vi "Teleop.vi"(10 "Match Info":T1={"Autonomous Elapsed Seconds"=0.0, "TeleOp Elapsed Seconds"=0.0, "Disabled Elapsed Seconds"=0.0, "Visited Autonomous"=FALSE, "Visited TeleOp"=FALSE, "Visited Disabled"=FALSE, "Autonomous Settings"={"Autonomous Style"=enum."Independent", "VI Refnum"=refnum}}, 11 "Call Context":T2) -> ()   [LabVIEW 2020]
doc: "This VI is called for each TeleOp packet received from the DS where the robot is not disabled. It is often used to read from the joysticks and update I/O or to update setpoints for timed control loops. It should complete and return within 20 milliseconds or it may miss DS packets."
uses:
  <vilib>/Rock Robotics/WPI/DriverStation/WPI_DriverStationDerivedRobotMode.ctl
  <vilib>/Rock Robotics/WPI/DriverStation/WPI_DriverStationMatch Info.ctl
  <vilib>/Rock Robotics/WPI/Utilities/WPI_GetSetVariantRefNum.vi
  <vilib>/Rock Robotics/Network Tables/NT Read Boolean.vi
  <vilib>/Rock Robotics/Network Tables/NT Read Number.vi
  Variable BX.vi
  RX.vi
  LX.vi
panel:
  out "Sample Slider 0":dbl(slide) scale=0.0..5.0
  out "Sample Boolean 1":bool
  out "Sample Boolean 0":bool
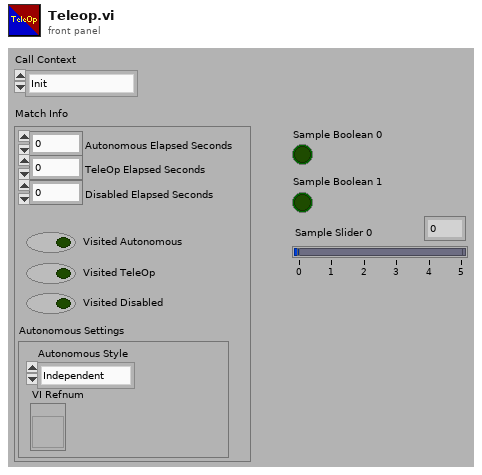
[diagram p1: front panel]
types:
  T1 = typedef "WPI_DriverStationMatch Info.ctl" = cluster{"Autonomous Elapsed Seconds":dbl, "TeleOp Elapsed Seconds":dbl, "Disabled Elapsed Seconds":dbl, "Visited Autonomous":bool, "Visited TeleOp":bool, "Visited Disabled":bool, "Autonomous Settings":cluster{"Autonomous Style":enum16{"Iterative", "Independent"}, "VI Refnum":refnum<vi>}}
  T2 = typedef "WPI_DriverStationDerivedRobotMode.ctl" = enum16{"Init", "Execute", "Stop"}
  T3 = typedef "WPI_MotorControlDeviceRef.ctl" = cluster{"DeviceStatus":errorcluster, "Type":T4, "PWM":cluster{"PWM Channel":T5, "DeadBand":T6}, "CAN":cluster{"Device Number":u8, "SetOutput VI Ref":variant, "GetOutput VI Ref":variant, "Enable VI Ref":variant, "Disable VI Ref":variant, "Data":variant}, "Invert":bool, "DIO PWM":cluster{"PWM \"Enable\" Channel":T5, "DIOChannel":T7, "PWM Rate":dbl}}
  T4 = typedef "WPI_MotorControlType.ctl" = enum16{"PWM", "CAN", "DIO PWM"}
  T5 = typedef "FPGA_DIOPWMChannel.ctl" = enum8{"PWM 0", "PWM 1", "PWM 2", "PWM 3", "PWM 4", "PWM 5", "PWM 6", "PWM 7", "PWM 8", "PWM 9", "PWM MXP 0", "PWM MXP 1", "PWM MXP 2", "PWM MXP 3", "PWM MXP 4", "PWM MXP 5", "PWM MXP 6", "PWM MXP 7", "PWM MXP 8", "PWM MXP 9", "Invalid"}
  T6 = typedef "WPI_PWMDeadband.ctl" = cluster{"Name":string, "maxPositivePwm":i32, "minPositivePwm":i32, "centerPwm":i32, "maxNegativePwm":i32, "minNegativePwm":i32, "angularRange":u16}
  T7 = typedef "FPGA_DIOChannel.ctl" = enum8{"DIO 0", "DIO 1", "DIO 2", "DIO 3", "DIO 4", "DIO 5", "DIO 6", "DIO 7", "DIO 8", "DIO 9", "DIO MXP 0", "DIO MXP 1", "DIO MXP 2", "DIO MXP 3", "DIO MXP 4", "DIO MXP 5", "DIO MXP 6", "DIO MXP 7", "DIO MXP 8", "DIO MXP 9", "DIO MXP 10", "DIO MXP 11", "DIO MXP 12", "DIO MXP 13", "DIO MXP 14", "DIO MXP 15", "SPI Port CS1", "SPI Port CS2", "SPI Port CS3", "SPI Port MISO", "SPI Port MOSI", "Invalid"}
  T8 = typedef "WPI_JoystickDevRef.ctl" = cluster{"Device":T9}
  T9 = typedef "WPI_JoystickDeviceEnum.ctl" = enum16{"USB 0", "USB 1", "USB 2", "USB 3", "USB 4", "USB 5"}
  T10 = typedef "WPI_RobotDriveDevRef.ctl" = cluster{"DevStatus":errorcluster, "Motors[]":T3[], "Square Inputs":bool, "Max Output":dbl}
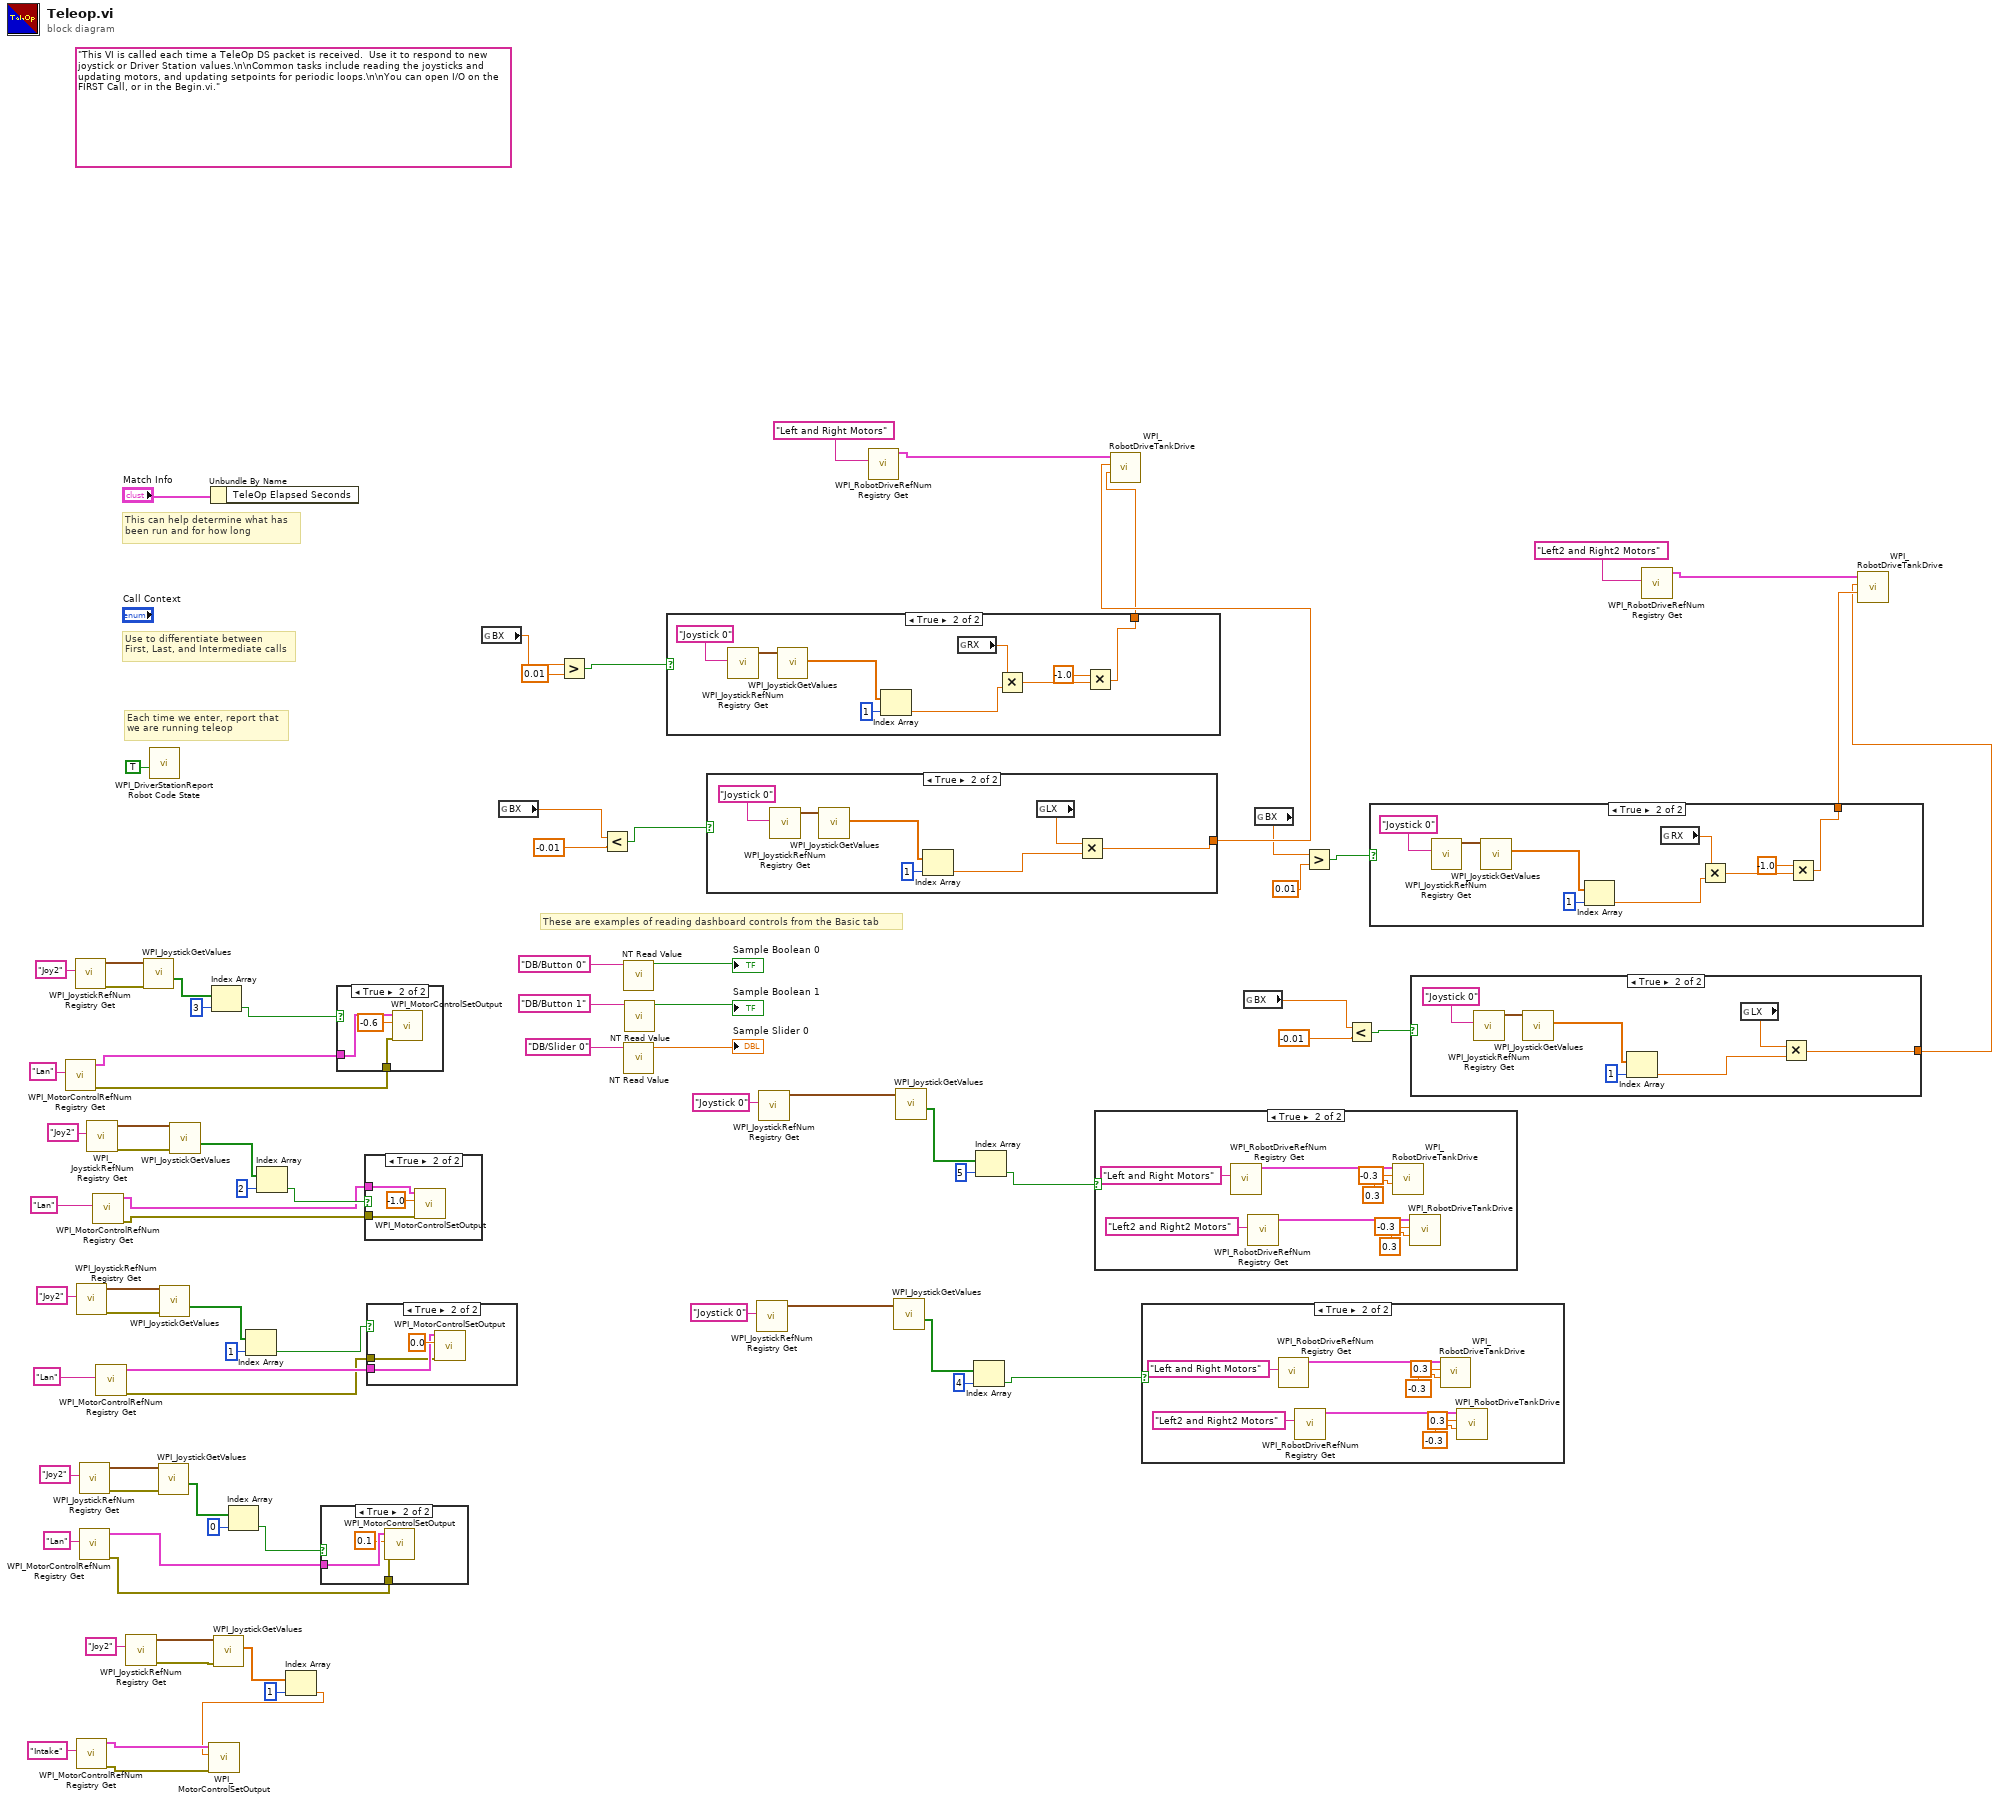
[diagram p0: block diagram]
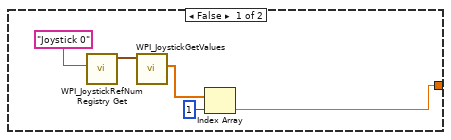
[diagram p8: hidden frame]
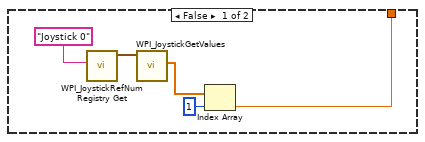
[diagram p9: hidden frame]
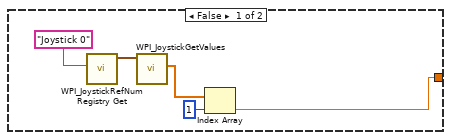
[diagram p10: hidden frame]
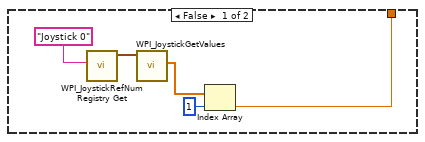
[diagram p11: hidden frame]
diagram:
  (unwired) "This VI is called each time a TeleOp DS packet is received.  Use it to respond to new joystick or Driver Station values.\n\nCommon tasks include reading the joysticks and updating motors, and updating setpoints for periodic loops.\n\nYou can open I/O on the FIRST Call, or in the Begin.vi."
  # "These are examples of reading dashboard controls from the Basic tab"
  # "Each time we enter, report that\nwe are running teleop"
  # "Use to differentiate between\nFirst, Last, and Intermediate calls"
  # "This can help determine what has\nbeen run and for how long"
  n1 = call <vilib>:"WPI_MotorControlRefNum Registry Get.vi"("refnum name"="Lan") -> ("error out"=w10:errorcluster, "MotorControlDevRef"=w11:T3)  [unwired: 9 in]
  n2 = call <vilib>:"WPI_JoystickRefNum Registry Get.vi"("refnum name"="Joy2") -> ("error out"=w15:errorcluster, "JoystickDevRef"=w16:T8)  [unwired: 9 in]
  n3 = call <vilib>:"WPI_JoystickRefNum Registry Get.vi"("refnum name"="Joy2") -> ("error out"=w34:errorcluster, "JoystickDevRef"=w35:T8)  [unwired: 9 in]
  n4 = call <vilib>:"WPI_MotorControlRefNum Registry Get.vi"("refnum name"="Intake") -> ("error out"=w23:errorcluster, "MotorControlDevRef"=w24:T3)  [unwired: 9 in]
  n5 = call <vilib>:"WPI_JoystickRefNum Registry Get.vi"("refnum name"="Joy2") -> ("error out"=w6:errorcluster, "JoystickDevRef"=w7:T8)  [unwired: 9 in]
  n6 = call <vilib>:"WPI_MotorControlRefNum Registry Get.vi"("refnum name"="Lan") -> ("error out"=w1:errorcluster, "MotorControlDevRef"=w2:T3)  [unwired: 9 in]
  n7 = call <vilib>:"WPI_JoystickRefNum Registry Get.vi"("refnum name"="Joy2") -> ("error out"=w43:errorcluster, "JoystickDevRef"=w44:T8)  [unwired: 9 in]
  n8 = call <vilib>:"WPI_MotorControlRefNum Registry Get.vi"("refnum name"="Lan") -> ("error out"=w38:errorcluster, "MotorControlDevRef"=w37:T3)  [unwired: 9 in]
  n9 = call <vilib>:"WPI_MotorControlRefNum Registry Get.vi"("refnum name"="Lan") -> ("error out"=w28:errorcluster, "MotorControlDevRef"=w29:T3)  [unwired: 9 in]
  n10 = call <vilib>:"WPI_JoystickRefNum Registry Get.vi"("refnum name"="Joy2") -> ("error out"=w25:errorcluster, "JoystickDevRef"=w26:T8)  [unwired: 9 in]
  n11 = call <vilib>:"WPI_JoystickGetValues.vi"("error in (no error)"=w15, "JoystickDevRef"=w16) -> ("Buttons"=w14:bool[])  [unwired: 5 in, 4 out]
  n12 = call <vilib>:"WPI_DriverStationReport Robot Code State.vi"("TeleOp"=TRUE ("Autonomous")) -> ()  [unwired: 10 in, 1 out]
  n13 = call <vilib>:"WPI_JoystickGetValues.vi"("error in (no error)"=w6, "JoystickDevRef"=w7) -> ("Buttons"=w5:bool[])  [unwired: 5 in, 4 out]
  n14 = call <vilib>:"WPI_JoystickGetValues.vi"("error in (no error)"=w34, "JoystickDevRef"=w35) -> ("Buttons"=w33:bool[])  [unwired: 5 in, 4 out]
  n15 = call <vilib>:"WPI_JoystickGetValues.vi"("error in (no error)"=w43, "JoystickDevRef"=w44) -> ("Buttons"=w41:bool[])  [unwired: 5 in, 4 out]
  n16 = Unbundle By Name("Match Info") -> ()  [unwired: 1 out]
  n17 = Index Array(array=w14, index=3) -> (element=w12:bool)
  n18 = call <vilib>:"WPI_JoystickGetValues.vi"("error in (no error)"=w25, "JoystickDevRef"=w26) -> ("Axes"=w22:dbl[])  [unwired: 5 in, 4 out]
  n19 = Index Array(array=w5, index=0) -> (element=w3:bool)
  n20 = Index Array(array=w33, index=1) -> (element=w31:bool)
  n21 = Index Array(array=w41, index=2) -> (element=w40:bool)
  n22 = Index Array(array=w22, index=1) -> (element=w21:dbl)
  n23 = call <vilib>:"WPI_MotorControlSetOutput.vi"("error in (no error)"=w23, "Output"=w21, "MotorControlDevRef"=w24) -> ()  [unwired: 6 in, 3 out]
  n24 = case shown="True" w3 {
    tunnel: w2 -> [_ w86]
    tunnel: w1 -> [_ w85]
    frame False {
    }
    frame True {
      n25 = call <vilib>:"WPI_MotorControlSetOutput.vi"("error in (no error)"=w85, "Output"=0.1, "MotorControlDevRef"=w86) -> ()  [unwired: 6 in, 3 out]
    }
  }
  n26 = case shown="True" w12 {
    tunnel: w11 -> [_ w89]
    tunnel: w10 -> [_ w88]
    frame False {
    }
    frame True {
      n27 = call <vilib>:"WPI_MotorControlSetOutput.vi"("error in (no error)"=w88, "Output"=-0.6, "MotorControlDevRef"=w89) -> ()  [unwired: 6 in, 3 out]
    }
  }
  n28 = case shown="True" w40 {
    tunnel: w38 -> [_ w91]
    tunnel: w37 -> [_ w90]
    frame False {
    }
    frame True {
      n29 = call <vilib>:"WPI_MotorControlSetOutput.vi"("error in (no error)"=w91, "Output"=-1.0, "MotorControlDevRef"=w90) -> ()  [unwired: 6 in, 3 out]
    }
  }
  n30 = case shown="True" w31 {
    tunnel: w29 -> [_ w94]
    tunnel: w28 -> [_ w93]
    frame False {
    }
    frame True {
      n31 = call <vilib>:"WPI_MotorControlSetOutput.vi"("error in (no error)"=w93, "Output"=0.0, "MotorControlDevRef"=w94) -> ()  [unwired: 6 in, 3 out]
    }
  }
  n32 = global read "Variable BX.vi" "BX"() -> (w73:dbl)
  n33 = global read "Variable BX.vi" "BX"() -> (w70:dbl)
  n34 = Greater?(x=w73, y=0.01) -> (0:w71:bool)
  n35 = Less?(x=w70, y=-0.01) -> (x < y?=w68:bool)
  n36 = call-poly <vilib>:"NT Read Value.vi"("Name"="DB/Button 0" ("refnum name")) -> ("Boolean"=→"Sample Boolean 0":bool)  [unwired: 9 in, 1 out]
  n37 = call-poly <vilib>:"NT Read Value.vi"("Name"="DB/Slider 0" ("refnum name")) -> ("Numeric"=→"Sample Slider 0":dbl)  [unwired: 9 in, 1 out]
  n38 = call-poly <vilib>:"NT Read Value.vi"("Name"="DB/Button 1" ("refnum name")) -> ("Boolean"=→"Sample Boolean 1":bool)  [unwired: 9 in, 1 out]
  n39 = case shown="True" w71 {
    tunnel: [w96 w101] -> w64
    frame False {
      n40 = call <vilib>:"WPI_JoystickRefNum Registry Get.vi"("refnum name"="Joystick 0") -> ("JoystickDevRef"=w99:T8)  [unwired: 1 in, 9 out]
      n41 = call <vilib>:"WPI_JoystickGetValues.vi"("JoystickDevRef"=w99) -> ("Axes"=w100:dbl[])  [unwired: 6 in, 4 out]
      n42 = Index Array(array=w100, index=1) -> (element=w96:dbl)
    }
    frame True {
      n43 = call <vilib>:"WPI_JoystickRefNum Registry Get.vi"("refnum name"="Joystick 0") -> ("JoystickDevRef"=w107:T8)  [unwired: 1 in, 9 out]
      n44 = call <vilib>:"WPI_JoystickGetValues.vi"("JoystickDevRef"=w107) -> ("Axes"=w105:dbl[])  [unwired: 6 in, 4 out]
      n45 = Index Array(array=w105, index=1) -> (element=w104:dbl)
      n46 = global read "RX.vi" "RX"() -> (w108:dbl)
      n47 = Multiply(x=w108, y=w104) -> (x*y=w103:dbl)
      n48 = Multiply(x=-1.0, y=w103) -> (x*y=w101:dbl)
    }
  }
  n49 = case shown="True" w68 {
    tunnel: [w110 w115] -> w65
    frame False {
      n50 = call <vilib>:"WPI_JoystickRefNum Registry Get.vi"("refnum name"="Joystick 0") -> ("JoystickDevRef"=w113:T8)  [unwired: 1 in, 9 out]
      n51 = call <vilib>:"WPI_JoystickGetValues.vi"("JoystickDevRef"=w113) -> ("Axes"=w114:dbl[])  [unwired: 6 in, 4 out]
      n52 = Index Array(array=w114, index=1) -> (element=w110:dbl)
    }
    frame True {
      n53 = call <vilib>:"WPI_JoystickRefNum Registry Get.vi"("refnum name"="Joystick 0") -> ("JoystickDevRef"=w120:T8)  [unwired: 1 in, 9 out]
      n54 = call <vilib>:"WPI_JoystickGetValues.vi"("JoystickDevRef"=w120) -> ("Axes"=w118:dbl[])  [unwired: 6 in, 4 out]
      n55 = Index Array(array=w118, index=1) -> (element=w116:dbl)
      n56 = global read "LX.vi" "LX"() -> (w117:dbl)
      n57 = Multiply(x=w117, y=w116) -> (x*y=w115:dbl)
    }
  }
  n58 = call <vilib>:"WPI_JoystickRefNum Registry Get.vi"("refnum name"="Joystick 0") -> ("JoystickDevRef"=w54:T8)  [unwired: 9 in, 1 out]
  n59 = call <vilib>:"WPI_JoystickRefNum Registry Get.vi"("refnum name"="Joystick 0") -> ("JoystickDevRef"=w50:T8)  [unwired: 9 in, 1 out]
  n60 = call <vilib>:"WPI_RobotDriveRefNum Registry Get.vi"("refnum name"="Left and Right Motors") -> ("RobotDriveDevRef"=w74:T10)  [unwired: 1 in, 9 out]
  n61 = call <vilib>:"WPI_JoystickGetValues.vi"("JoystickDevRef"=w54) -> ("Buttons"=w53:bool[])  [unwired: 6 in, 4 out]
  n62 = call <vilib>:"WPI_JoystickGetValues.vi"("JoystickDevRef"=w50) -> ("Buttons"=w49:bool[])  [unwired: 6 in, 4 out]
  n63 = Index Array(array=w53, index=4) -> (element=w46:bool)
  n64 = Index Array(array=w49, index=5) -> (element=w47:bool)
  n65 = case shown="True" w47 {
    frame False {
    }
    frame True {
      n66 = call <vilib>:"WPI_RobotDriveRefNum Registry Get.vi"("refnum name"="Left and Right Motors") -> ("RobotDriveDevRef"=w129:T10)  [unwired: 9 in, 1 out]
      n67 = call <vilib>:"WPI_RobotDriveRefNum Registry Get.vi"("refnum name"="Left2 and Right2 Motors") -> ("RobotDriveDevRef"=w128:T10)  [unwired: 9 in, 1 out]
      n68 = call <vilib>:"WPI_RobotDriveTankDrive.vi"("Right axis value"=0.3, "Left axis value"=-0.3, "RobotDriveDevRef"=w129) -> ()  [unwired: 6 in, 3 out]
      n69 = call <vilib>:"WPI_RobotDriveTankDrive.vi"("Right axis value"=0.3, "Left axis value"=-0.3, "RobotDriveDevRef"=w128) -> ()  [unwired: 6 in, 3 out]
    }
  }
  n70 = call <vilib>:"WPI_RobotDriveTankDrive.vi"("Right axis value"=w64, "Left axis value"=w65, "RobotDriveDevRef"=w74) -> ()  [unwired: 6 in, 3 out]
  n71 = case shown="True" w46 {
    frame False {
    }
    frame True {
      n72 = call <vilib>:"WPI_RobotDriveRefNum Registry Get.vi"("refnum name"="Left and Right Motors") -> ("RobotDriveDevRef"=w137:T10)  [unwired: 9 in, 1 out]
      n73 = call <vilib>:"WPI_RobotDriveRefNum Registry Get.vi"("refnum name"="Left2 and Right2 Motors") -> ("RobotDriveDevRef"=w136:T10)  [unwired: 9 in, 1 out]
      n74 = call <vilib>:"WPI_RobotDriveTankDrive.vi"("Right axis value"=-0.3, "Left axis value"=0.3, "RobotDriveDevRef"=w137) -> ()  [unwired: 6 in, 3 out]
      n75 = call <vilib>:"WPI_RobotDriveTankDrive.vi"("Right axis value"=-0.3, "Left axis value"=0.3, "RobotDriveDevRef"=w136) -> ()  [unwired: 6 in, 3 out]
    }
  }
  n76 = global read "Variable BX.vi" "BX"() -> (w60:dbl)
  n77 = global read "Variable BX.vi" "BX"() -> (w63:dbl)
  n78 = Greater?(x=w63, y=0.01) -> (0:w61:bool)
  n79 = Less?(x=w60, y=-0.01) -> (x < y?=w58:bool)
  n80 = case shown="True" w61 {
    tunnel: [w138 w143] -> w57
    frame False {
      n81 = call <vilib>:"WPI_JoystickRefNum Registry Get.vi"("refnum name"="Joystick 0") -> ("JoystickDevRef"=w141:T8)  [unwired: 1 in, 9 out]
      n82 = call <vilib>:"WPI_JoystickGetValues.vi"("JoystickDevRef"=w141) -> ("Axes"=w142:dbl[])  [unwired: 6 in, 4 out]
      n83 = Index Array(array=w142, index=1) -> (element=w138:dbl)
    }
    frame True {
      n84 = call <vilib>:"WPI_JoystickRefNum Registry Get.vi"("refnum name"="Joystick 0") -> ("JoystickDevRef"=w149:T8)  [unwired: 1 in, 9 out]
      n85 = call <vilib>:"WPI_JoystickGetValues.vi"("JoystickDevRef"=w149) -> ("Axes"=w147:dbl[])  [unwired: 6 in, 4 out]
      n86 = Index Array(array=w147, index=1) -> (element=w146:dbl)
      n87 = global read "RX.vi" "RX"() -> (w150:dbl)
      n88 = Multiply(x=w150, y=w146) -> (x*y=w145:dbl)
      n89 = Multiply(x=-1.0, y=w145) -> (x*y=w143:dbl)
    }
  }
  n90 = case shown="True" w58 {
    tunnel: [w152 w157] -> w56
    frame False {
      n91 = call <vilib>:"WPI_JoystickRefNum Registry Get.vi"("refnum name"="Joystick 0") -> ("JoystickDevRef"=w155:T8)  [unwired: 1 in, 9 out]
      n92 = call <vilib>:"WPI_JoystickGetValues.vi"("JoystickDevRef"=w155) -> ("Axes"=w156:dbl[])  [unwired: 6 in, 4 out]
      n93 = Index Array(array=w156, index=1) -> (element=w152:dbl)
    }
    frame True {
      n94 = call <vilib>:"WPI_JoystickRefNum Registry Get.vi"("refnum name"="Joystick 0") -> ("JoystickDevRef"=w162:T8)  [unwired: 1 in, 9 out]
      n95 = call <vilib>:"WPI_JoystickGetValues.vi"("JoystickDevRef"=w162) -> ("Axes"=w160:dbl[])  [unwired: 6 in, 4 out]
      n96 = Index Array(array=w160, index=1) -> (element=w158:dbl)
      n97 = global read "LX.vi" "LX"() -> (w159:dbl)
      n98 = Multiply(x=w159, y=w158) -> (x*y=w157:dbl)
    }
  }
  n99 = call <vilib>:"WPI_RobotDriveRefNum Registry Get.vi"("refnum name"="Left2 and Right2 Motors") -> ("RobotDriveDevRef"=w66:T10)  [unwired: 1 in, 9 out]
  n100 = call <vilib>:"WPI_RobotDriveTankDrive.vi"("Right axis value"=w57, "Left axis value"=w56, "RobotDriveDevRef"=w66) -> ()  [unwired: 6 in, 3 out]
